vi "Read SBOM Components from VIPC File.vi"(8 "error in (no error)":errorcluster, 11 "VIPC path":path) -> (0 "error out":errorcluster, 3 "SBOM Components out":refnum<class "CycloneDX Component.lvclass">[](array[class]))   [LabVIEW 2017, in "VIP SBOM Support.lvlib"]
doc: "Converts a package list from a VIPC file into a list of CycloneDX SBOM components."
uses:
  VIP SBOM Support.lvlib
  CycloneDX/CycloneDX Component/CycloneDX Component.lvclass
  <vilib>/JKI/VIPM API/VIPM API_vipm_api.lvlib
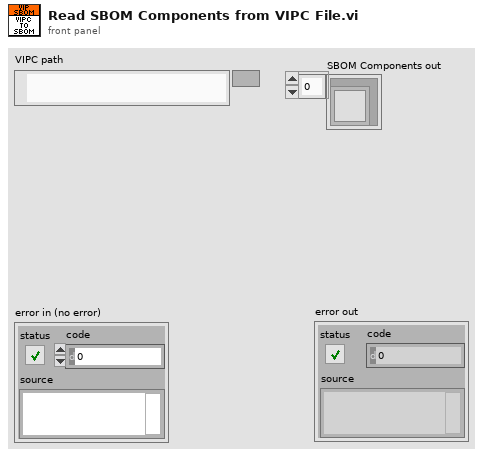
[diagram p1: front panel]
types:
  T1 = typedef "VIPM API_vipm_api.lvlib/Library Contents Cluster_vipm_api.ctl" = cluster{"Package Name":string, "Version":string, "Display Name":string, "Repository Name":string, "Company Name":string, "License Type":string, "Installed":bool, "Deprecated":bool, "Dependency or Conflict Problem":bool, "Downloaded":bool}
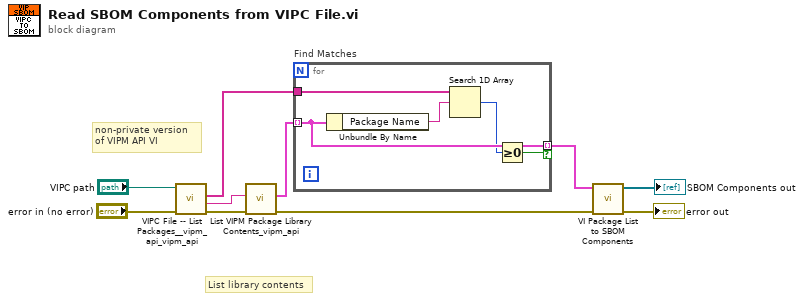
[diagram p0: block diagram]
diagram:
  # "List library contents"
  # "non-private version of VIPM API VI"
  n1 = call "VIPC File -- List Packages__vipm_api_vipm_api.vi"("error in (no error)"="error in (no error)", "VIPC File Path"="VIPC path") -> ("error out"=w9:errorcluster, "VIPC LabVIEW Version"=w7:string, "Package List"=w8:string[])  [unwired: 6 in, 1 out]
  n2 = call <vilib>:"List VIPM Package Library Contents_vipm_api.vi"("error in (no error)"=w9, "LabVIEW Version"=w7) -> ("error out"=w4:errorcluster, "Library Contents []"=w10:T1[])  [unwired: 8 in]
  n3 = for "Find Matches" {
    tunnel: w10 -> [w15] mode=indexing
    tunnel: w8 -> [w14]
    tunnel: [w15] -> w5 mode=indexing if=w12
    n4 = Unbundle By Name(w15) -> ("Package Name"=w13:string)
    n5 = Search 1D Array(1D array=w14, element=w13) -> (index of element=w11:i32)  [unwired: 1 in]
    n6 = Greater Or Equal To 0?(x=w11) -> (x >= 0?=w12:bool)
  }
  n7 = call "VI Package List to SBOM Components.vi"("error in (no error)"=w4, "VIP List in"=w5) -> ("error out"=→"error out":errorcluster, "SBOM Components out"=→"SBOM Components out":refnum<class "CycloneDX Component.lvclass">[])  [unwired: 8 in]
